vi "Interprete message.vi"(8 "error in (no error)":errorcluster, 11 "TCS_ACS in":refnum<class "Header content.lvclass">) -> (0 "error out":errorcluster, 3 "TCS_ACS out":refnum<class "Header content.lvclass">)   [LabVIEW 2018, in "Header content.lvclass"]
doc: "Verify the JSON sent by the control interface"
uses:
  Header content.lvclass
  Header content.lvclass/Header content.ctl
panel:
  in  "Header data":T1
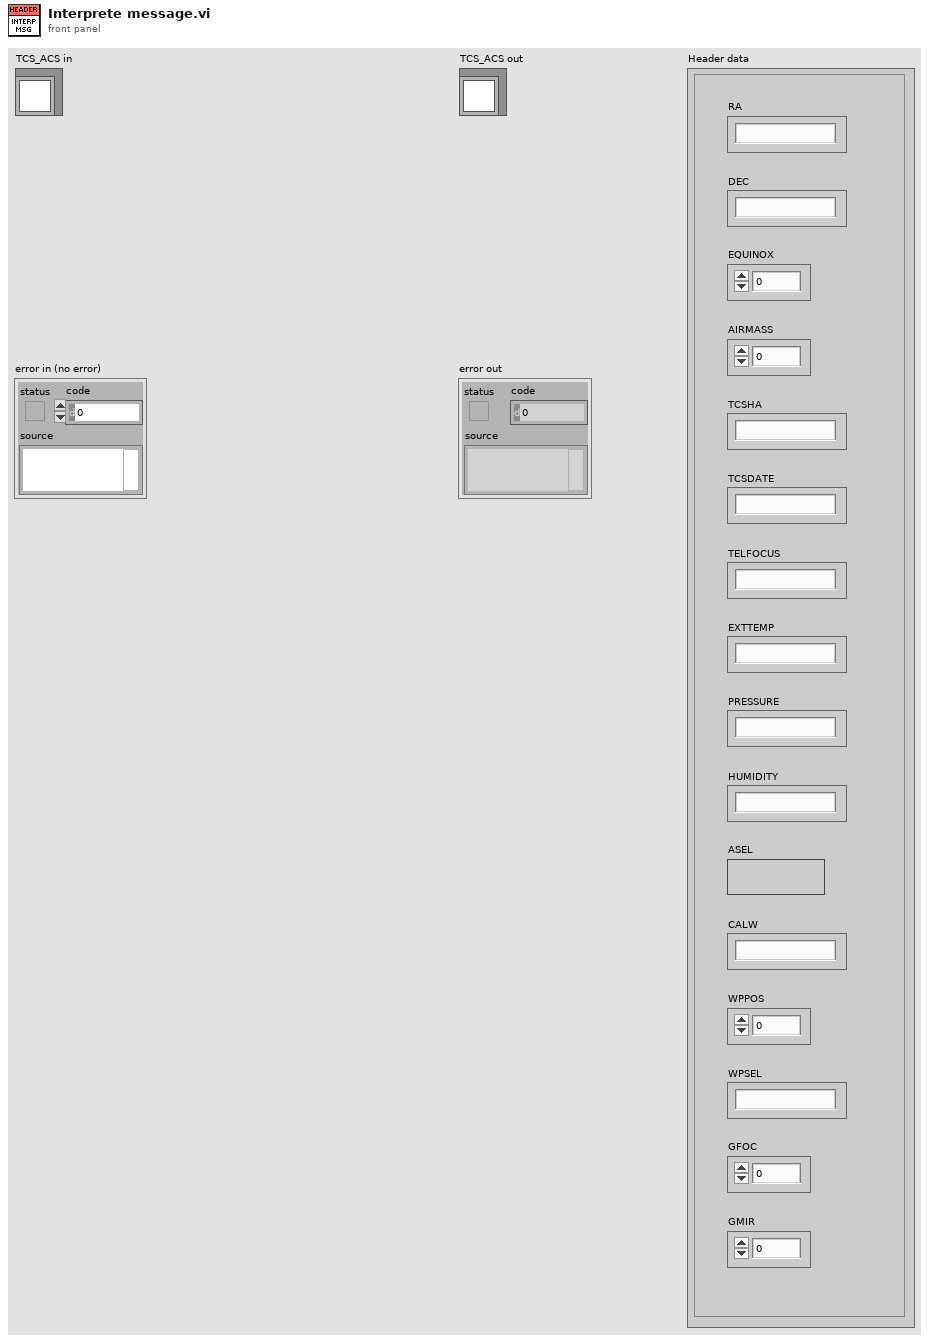
[diagram p1: front panel]
types:
  T1 = cluster{"RA":string, "DEC":string, "EQUINOX":dbl, "AIRMASS":dbl, "TCSHA":string, "TCSDATE":string, "TELFOCUS":string, "EXTTEMP":string, "PRESSURE":string, "HUMIDITY":string, "ASEL":bool, "CALW":string, "WPPOS":u16, "WPSEL":string, "GFOC":u16, "GMIR":u16}
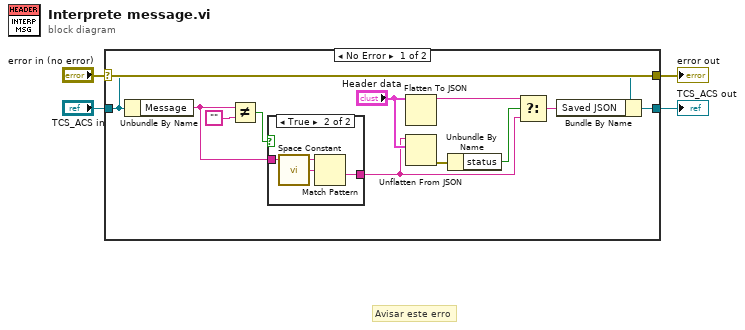
[diagram p0: block diagram]
diagram:
  # "Avisar este erro"
  n1 = case shown="No Error" "error in (no error)" {
    selector: "error in (no error)" -> [w13 w21]
    tunnel: [w13 w21] -> w3
    tunnel: [w11 w20] -> w1
    tunnel: "TCS_ACS in" -> [w12 w20]
    frame No Error {
      n2 = Unbundle By Name(w12) -> ("Message"=w14:string)
      n3 = Not Equal?(x=w14, y="") -> (x != y?=w15:bool)
      n4 = case shown="True" w15 {
        tunnel: w14 -> [_ w18]
        tunnel: [_ w17] -> w6
        frame False {
        }
        frame True {
          n5 = call <vilib>:"Space Constant.vi"() -> ("String"=w19:string)
          n6 = Match Pattern(string=w18, regular expression=w19) -> (after substring=w17:string)  [unwired: 1 in, 3 out]
        }
      }
      n7 = Flatten To JSON(anything="Header data") -> (JSON string=w7:string)  [unwired: 2 in, 1 out]
      n8 = Unflatten From JSON(JSON string=w6, type and defaults="Header data") -> (error out=w9:errorcluster)  [unwired: 5 in, 1 out]
      n9 = Unbundle By Name(w9) -> ("status"=w8:bool)
      n10 = Select(t=w7, s=w8, f=w6) -> (s? t:f=w5:string)
      n11 = Bundle By Name(cluster=w12, "Saved JSON"=w5) -> (w11:refnum<class "Header content.lvclass">)
    }
    frame Error {
    }
  }
  "error out" <- w3
  "TCS_ACS out" <- w1
